vi "根据当前状态选择下一状态.vi"(0 "测试项目队列输入":refnum<queue>, 1 "当前状态":T2=enum."指令测试") -> (2 "测试项目队列输出":refnum<queue>, 3 "切换卡片界面名称":T1=enum."初始化配置", 4 "下一状态":T2=enum."指令测试")   [LabVIEW 2015]
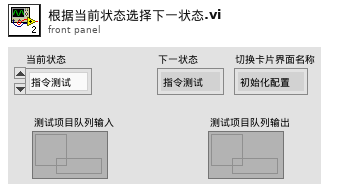
[diagram p1: front panel]
types:
  T1 = typedef "切换卡片界面名称.ctl" = enum32{"主界面", "初始化配置", "指令测试", "数据测试", "特殊功能测试", "心跳包测试", "升级测试", "中心切换测试", "生成报告"}
  T2 = typedef "状态机状态.ctl" = enum16{"初始化", "等待按键", "串口操作", "检索模块", "网络测试", "测试项目", "模块参数配置", "指令测试", "数据测试", "特殊功能测试", "心跳包测试", "升级测试", "中心切换测试", "计算测试耗时", "生成报告", "提示消息", "退出"}
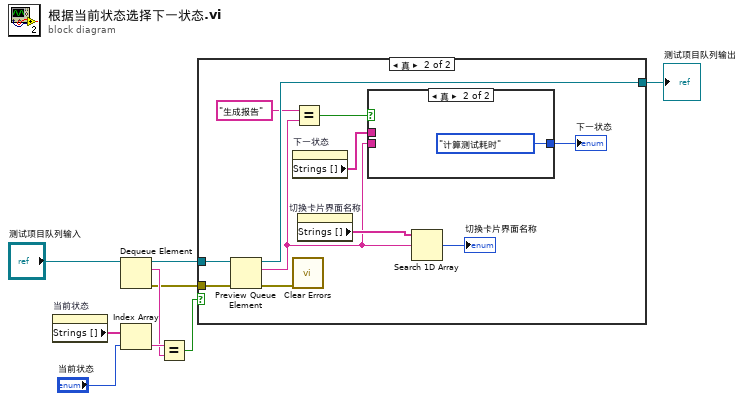
[diagram p0: block diagram]
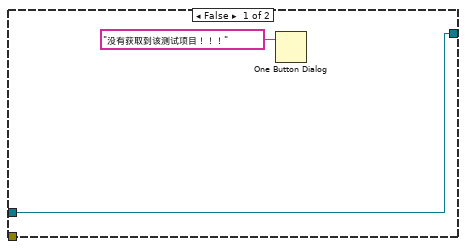
[diagram p2: hidden frame]
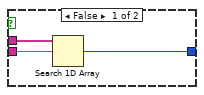
[diagram p3: hidden frame]
diagram:
  n1 = property on="当前状态" class="Enum (严格)"() -> ("Strings []"=w9:string[])  [unwired: 2 in, 2 out]
  n2 = Dequeue Element(queue="测试项目队列输入") -> (queue out=w3:refnum<queue>, element=w4:string, error out=w1:errorcluster)  [unwired: 2 in, 1 out]
  n3 = Index Array(array=w9, index="当前状态") -> (element=w6:string)
  n4 = Equal?(x=w6, y=w4) -> (x = y?=w8:bool)
  n5 = case shown="真" w8 {
    tunnel: w3 -> [w10 w22]
    tunnel: [w10 w21] -> w2
    tunnel: w1 -> [_ w13]
    frame False {
      n6 = One Button Dialog(message="没有获取到该测试项目！！！" ("消息")) -> ()  [unwired: 1 in, 1 out]
    }
    frame True {
      n7 = Preview Queue Element(queue=w22, error in (no error)=w13) -> (queue out=w21:refnum<queue>, element=w14:string, error out=w12:errorcluster)  [unwired: 1 in, 1 out]
      n8 = property on="下一状态" class="Enum (严格)"() -> ("Strings []"=w17:string[])  [unwired: 2 in, 2 out]
      n9 = call <vilib>:"Clear Errors.vi"("error in (no error)"=w12) -> ()  [unwired: 5 in, 2 out]
      n10 = Equal?(x="生成报告", y=w14) -> (x = y?=w15:bool)
      n11 = property on="切换卡片界面名称" class="Enum (严格)"() -> ("Strings []"=w20:string[])  [unwired: 2 in, 2 out]
      n12 = case shown="真" w15 {
        tunnel: [w25 状态机状态."计算测试耗时" ("下一状态")] -> w18
        tunnel: w17 -> [w24 _]
        tunnel: w14 -> [w23 _]
        frame False {
          n13 = Search 1D Array(1D array=w24, element=w23) -> (index of element=w25:i32)  [unwired: 1 in]
        }
        frame True {
        }
      }
      "下一状态" <- w18
      n14 = Search 1D Array(1D array=w20, element=w14) -> (index of element=→"切换卡片界面名称":i32)  [unwired: 1 in]
    }
  }
  "测试项目队列输出" <- w2
